vi "SV TDMS Convert Scalar Function Info to Unit Info.vi"(7 "Y-unit string override":string, 11 "scalar info in":T1={"scalar function type"=10, "scalar function subtype"=19, " x-dimension"=0} {"scalar function type" items=["Speed"=3, "Ratio"=6, "Count"=7, "-"=9, "Level"=10, "-"=19, "None"=98]; "scalar function subtype" items=["Value"=19, "DC"=11, "AC"=12, "RMS^2"=13, "RMS"=14, "Peak"=15, "Peak to peak"=16, "-"=20, "None"=98, "Unknown"=99]; "x-dimension" items=["Time (s)"=0, "Frequency-CB (Hz)"=1, "Frequency-CPB (Hz)"=1248, "Frequency-Arbitrary (Hz)"=2357, "Quefrency (s)"=2, "Revolutions (rev)"=3, "Order"=4, "Speed (RPM)"=11, "Speed (rad/s)"=21, "Critical Band"=31, "Critical Band Rate (Bark)"=32, "None"=98, "Index"=65535]}) -> (3 "unit info":T3)   [LabVIEW 2017]
doc: "Converts the X Dimension of scalar function info in into unit information."
uses:
  <vilib>/addons/_NISVFA/_Shared subVIs/Controls/svc_Unit Info.ctl
  <vilib>/addons/_NISVFA/_Shared subVIs/Controls/NI Scalar Function Info.ctl
  <vilib>/addons/_NISVFA/_Shared subVIs/Controls/svc_X-Axis Units.ctl
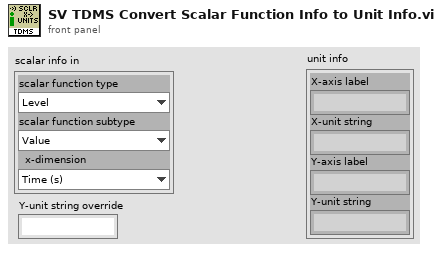
[diagram p1: front panel]
types:
  T1 = typedef "NI Scalar Function Info.ctl" = cluster{"scalar function type":u16, "scalar function subtype":u16, " x-dimension":T2}
  T2 = typedef "svc_X-Axis Units.ctl" = u16
  T3 = typedef "svc_Unit Info.ctl" = cluster{"X-axis label":string, "X-unit string":string, "Y-axis label":string, "Y-unit string":string}
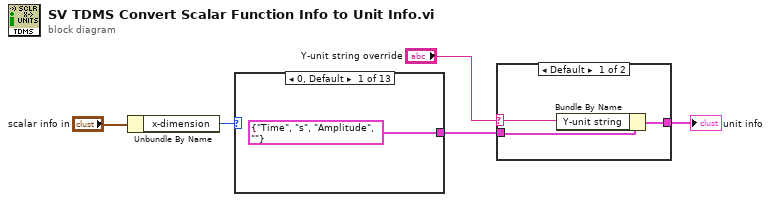
[diagram p0: block diagram]
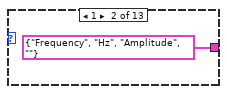
[diagram p3: hidden frame]
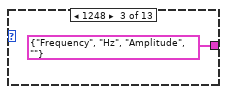
[diagram p4: hidden frame]
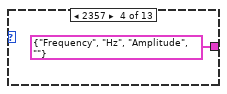
[diagram p5: hidden frame]
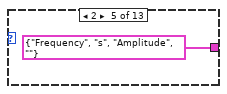
[diagram p6: hidden frame]
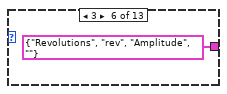
[diagram p7: hidden frame]
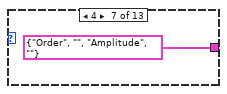
[diagram p8: hidden frame]
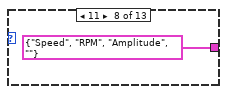
[diagram p9: hidden frame]
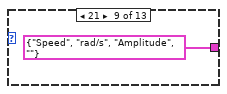
[diagram p10: hidden frame]
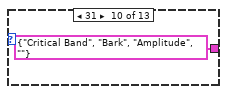
[diagram p11: hidden frame]
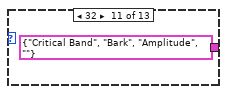
[diagram p12: hidden frame]
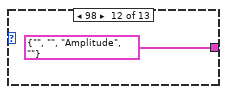
[diagram p13: hidden frame]
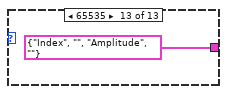
[diagram p14: hidden frame]
diagram:
  n1 = Unbundle By Name("scalar info in") -> ("x-dimension"=w5:T2)
  n2 = case shown="0, Default" w5 {
    tunnel: [T3 {"X-axis label"="Time", "X-unit string"="s", "Y-axis label"="Amplitude", "Y-unit string"=""} ("unit info") T3 {"X-axis label"="Frequency", "X-unit string"="Hz", "Y-axis label"="Amplitude", "Y-unit string"=""} ("unit info") T3 {"X-axis label"="Frequency", "X-unit string"="Hz", "Y-axis label"="Amplitude", "Y-unit string"=""} ("unit info") T3 {"X-axis label"="Frequency", "X-unit string"="Hz", "Y-axis label"="Amplitude", "Y-unit string"=""} ("unit info") T3 {"X-axis label"="Frequency", "X-unit string"="s", "Y-axis label"="Amplitude", "Y-unit string"=""} ("unit info") T3 {"X-axis label"="Revolutions", "X-unit string"="rev", "Y-axis label"="Amplitude", "Y-unit string"=""} ("unit info") T3 {"X-axis label"="Order", "X-unit string"="", "Y-axis label"="Amplitude", "Y-unit string"=""} ("unit info") T3 {"X-axis label"="Speed", "X-unit string"="RPM", "Y-axis label"="Amplitude", "Y-unit string"=""} ("unit info") T3 {"X-axis label"="Speed", "X-unit string"="rad/s", "Y-axis label"="Amplitude", "Y-unit string"=""} ("unit info") T3 {"X-axis label"="Critical Band", "X-unit string"="Bark", "Y-axis label"="Amplitude", "Y-unit string"=""} ("unit info") T3 {"X-axis label"="Critical Band", "X-unit string"="Bark", "Y-axis label"="Amplitude", "Y-unit string"=""} ("unit info") T3 {"X-axis label"="", "X-unit string"="", "Y-axis label"="Amplitude", "Y-unit string"=""} ("unit info") T3 {"X-axis label"="Index", "X-unit string"="", "Y-axis label"="Amplitude", "Y-unit string"=""} ("unit info")] -> w2
    frame 0, Default {
    }
    frame 1 {
    }
    frame 1248 {
    }
    frame 2357 {
    }
    frame 2 {
    }
    frame 3 {
    }
    frame 4 {
    }
    frame 11 {
    }
    frame 21 {
    }
    frame 31 {
    }
    frame 32 {
    }
    frame 98 {
    }
    frame 65535 {
    }
  }
  n3 = case shown="Default" "Y-unit string override" {
    selector: "Y-unit string override" -> [w20 _]
    tunnel: w2 -> [w21 w22]
    tunnel: [w19 w22] -> w1
    frame Default {
      n4 = Bundle By Name(cluster=w21, "Y-unit string"=w20) -> (w19:T3)
    }
    frame "" {
    }
  }
  "unit info" <- w1
